vi "QuadraticMagField.vi"() -> ()   [LabVIEW 2018]
uses:
  <vilib>/Native 3D Graph/xcontrol/3DPC_SurfacePlot.xctl
panel:
  in  "alpha":dbl
  out "3D Graph":refnum<class "Base Datatype.lvclass">[](xcontrol)
  in  "velocity":dbl
  out "zPosition":dbl
  out "xPosition":dbl
  out "vZfinal":dbl
  out "vXfinal":dbl
  out "vZinitial":dbl
  out "vXinitial":dbl
  out "yPosition":dbl
  out "vYfinal":dbl
  out "timeOfFlight":dbl format="%#_5g"
  in  "bField at Center":dbl
  in  "height":dbl
  out "vYinitial":dbl
  in  "eField":dbl
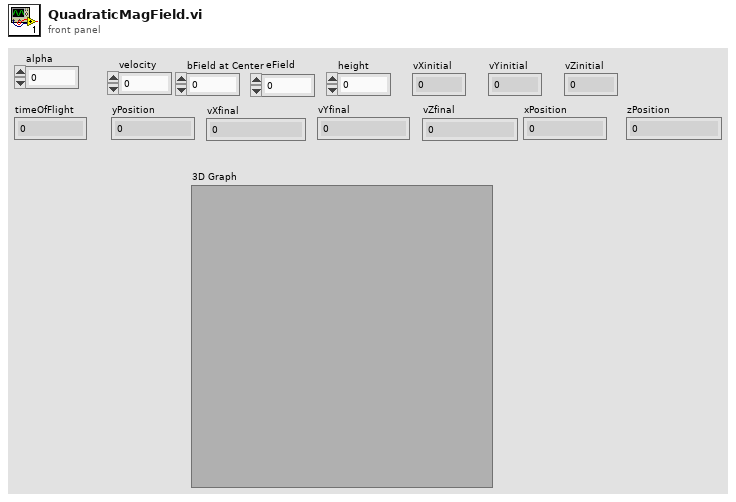
[diagram p1: front panel]
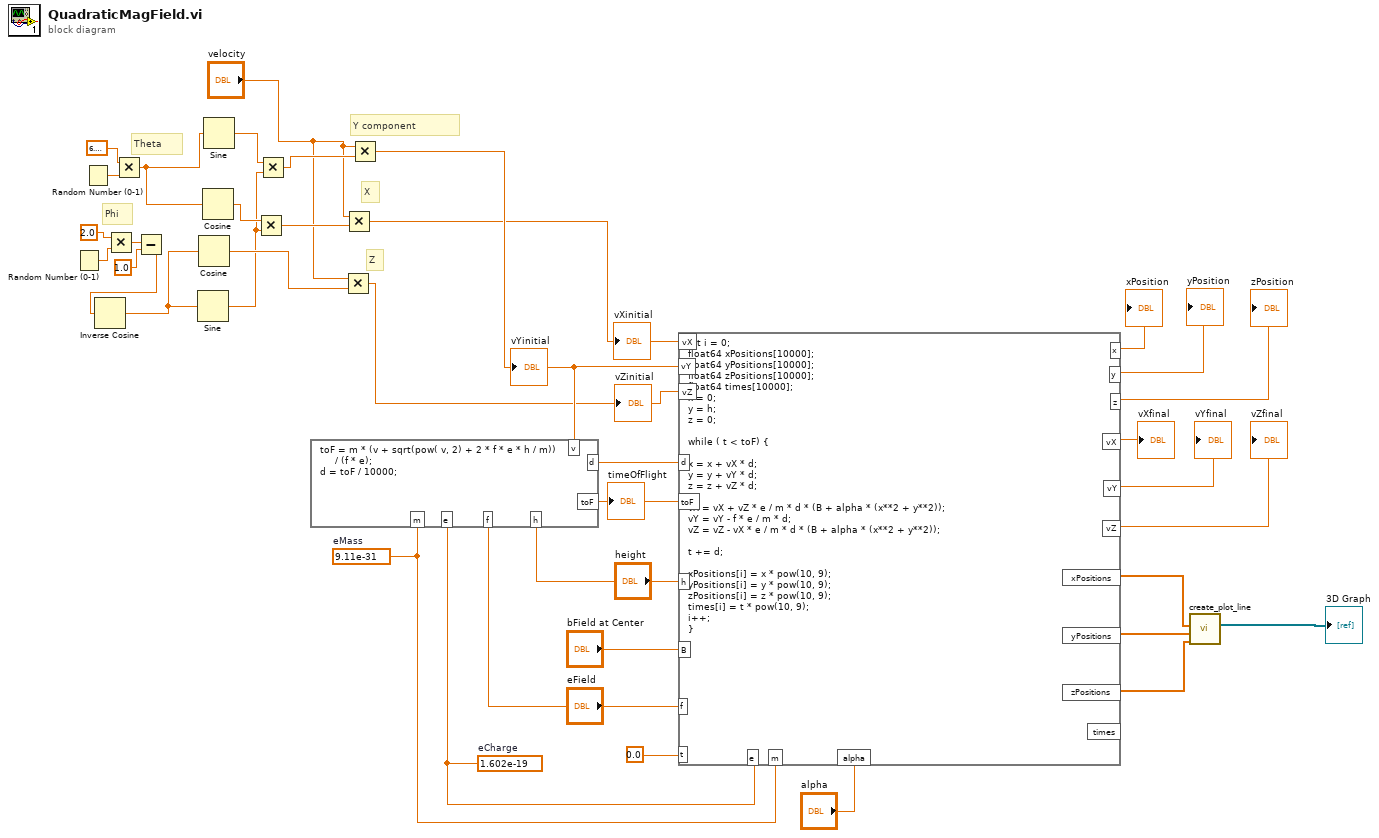
[diagram p0: block diagram]
diagram:
  w36 = 1.602e-19  # eCharge
  w35 = 9.11e-31  # eMass
  # "Phi"
  # "Theta"
  # "Z"
  # "X"
  # "Y component"
  n1 = Random Number (0-1)() -> (number: 0 to 1=w18:dbl)
  n2 = Random Number (0-1)() -> (number: 0 to 1=w21:dbl)
  n3 = Multiply(x=2.0, y=w18) -> (x*y=w17:dbl)
  n4 = Multiply(x=6.283185307179586, y=w21) -> (x*y=w15:dbl)
  n5 = Subtract(x=w17, y=1.0) -> (x-y=w14:dbl)
  n6 = Inverse Cosine(1:w14) -> (0:w13:dbl)
  n7 = Sine(x=w13) -> (sin(x)=w8:dbl)
  n8 = Cosine(x=w13) -> (cos(x)=w12:dbl)
  n9 = Cosine(x=w15) -> (cos(x)=w9:dbl)
  n10 = Sine(x=w15) -> (sin(x)=w11:dbl)
  n11 = Multiply(x=w9, y=w8) -> (x*y=w7:dbl)
  n12 = Multiply(x=w11, y=w8) -> (x*y=w10:dbl)
  n13 = Multiply(x="velocity", y=w12) -> (x*y=w4:dbl)
  "vZinitial" <- w4
  n14 = Multiply(x="velocity", y=w7) -> (x*y=w5:dbl)
  "vXinitial" <- w5
  n15 = Multiply(x="velocity", y=w10) -> (x*y=w6:dbl)
  "vYinitial" <- w6
  n16 = formula code="toF = m * (v + sqrt(pow( v, 2) + 2 * f * e * h / m))\n     / (f * e);\nd = toF / 10000;"("f"="eField", "h"="height", "v"=w6, "m"=w35, "e"=w36) -> ("toF"=w33:dbl, "d"=w34:dbl)
  "timeOfFlight" <- w33
  n17 = formula code="int i = 0;\nfloat64 xPositions[10000];\nfloat64 yPositions[10000];\nfloat64 zPositions[10000];\nfloat64 times[10000];\nx = 0;\ny = h;\nz = 0;\n\nwhile ( t < toF) {\n\nx = x + vX * d;\ny = y + vY * d;\nz = z + vZ * d;\n\nvX = vX + vZ * e / m * d * (B + alpha * (x**2 + y**2));\nvY = vY - f * e / m * d;\nvZ = vZ - vX * e / m * d * (B + alpha * (x**2 + y**2));\n\nt += d;\n\nxPositions[i] = x * pow(10, 9);\nyPositions[i] = y * pow(10, 9);\nzPositions[i] = z * pow(10, 9);\ntimes[i] = t * pow(10, 9);\ni++;\n}"("vY"=w6, "e"=w36, "m"=w35, "f"="eField", "d"=w34, "h"="height", "toF"=w33, "t"=0.0, "B"="bField at Center", "vX"=w5, "vZ"=w4, "alpha"="alpha") -> ("y"=→"yPosition":dbl, "vY"=→"vYfinal":dbl, "vX"=→"vXfinal":dbl, "vZ"=→"vZfinal":dbl, "x"=→"xPosition":dbl, "z"=→"zPosition":dbl, "xPositions"=w24:dbl[], "yPositions"=w23:dbl[], "zPositions"=w22:dbl[])  [unwired: 1 out]
  n18 = call <vilib>:"create_plot_line.vi"("z vector"=w22, "y vector"=w23, "x vector"=w24) -> ("plots out"=→"3D Graph":refnum<class "Base Datatype.lvclass">[])  [unwired: 2 in, 6 out]
